vi "Camera Stream.vi"() -> ()   [LabVIEW 2014]
doc: "This is a demonstration of opening and grabbing frames from a camera stream. Please check the block diagram for more information about the code."
uses:
  MSC Video_class/MSC Video.lvclass
  MSC Image_class/MSC Image.lvclass
panel:
  in  "CamID":i32
  out "error out":errorcluster
  in  "stop":bool
  out "Live Image":picture
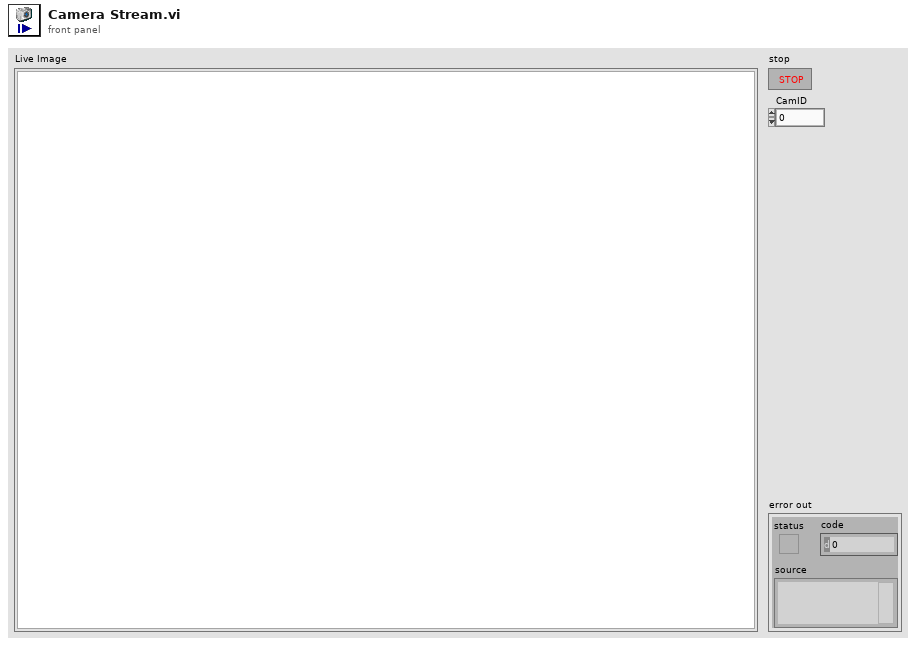
[diagram p1: front panel]
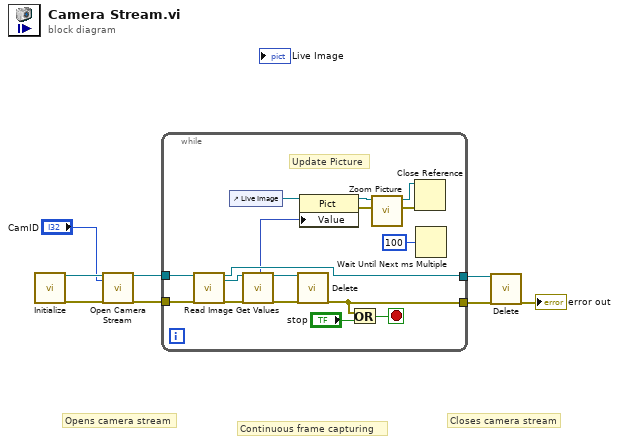
[diagram p0: block diagram]
diagram:
  # "Closes camera stream"
  # "Continuous frame capturing"
  # "Opens camera stream"
  n1 = call "Initialize.vi"() -> ("video out"=w8:refnum<class "MSC Video.lvclass">, "error out"=w7:errorcluster)  [unwired: 18 in]
  n2 = call-dynamic "Open Camera Stream.vi"("video in"=w8, "CamID"="CamID", "error in (no error)"=w7) -> ("video out"=w2:refnum<class "MSC Video.lvclass">, "error out"=w1:errorcluster)  [unwired: 15 in]
  n3 = while {
    tunnel: w2 -> [w25]
    tunnel: w1 -> [w24]
    tunnel: [w22] -> w6
    tunnel: [w16] -> w5
    stop <- w23 stop-if-true
    # "Update Picture"
    n4 = call-dynamic "Read Image.vi"("video in"=w25, "error in (no error)"=w24) -> ("video out"=w22:refnum<class "MSC Video.lvclass">, "image out"=w21:refnum<class "MSC Image.lvclass">, "error out"=w20:errorcluster)  [unwired: 15 in]
    n5 = control-ref of="Live Image"() -> (w15:refnum<vi>)
    n6 = call-dynamic "Get Values.vi"("image in"=w21, "error in (no error)"=w20) -> ("picture"=w10:picture, "image out"=w18:refnum<class "MSC Image.lvclass">, "error out"=w17:errorcluster)  [unwired: 10 in, 5 out]
    n7 = call-dynamic "Delete.vi"("image in"=w18, "error in (no error)"=w17) -> ("error out"=w16:errorcluster)  [unwired: 17 in]
    n8 = property class="Pict"(reference=w15, "Value"=w10) -> (reference out=w11:refnum<vi>, error out=w12:errorcluster)  [unwired: 1 in]
    n9 = Or(x=w16, y="stop") -> (x .or. y?=w23:bool)
    n10 = call "Zoom Picture.vi"("error in (no error)"=w12, "Picture in"=w11) -> ("error out"=w14:errorcluster, "Picture out"=w13:refnum<vi>)  [unwired: 8 in]
    n11 = Close Reference(reference=w13, error in (no error)=w14) -> ()  [unwired: 1 out]
    n12 = Wait Until Next ms Multiple(millisecond multiple=u32 100) -> ()  [unwired: 1 out]
  }
  n13 = call-dynamic "Delete.vi"("video in"=w6, "error in (no error)"=w5) -> ("error out"=→"error out":errorcluster)  [unwired: 17 in]
